vi "Release Session.vi"(0 "Session Handle":T1, 11 "error in (no error)":errorcluster, 13 "force destroy? (F)":bool) -> (15 "error out":errorcluster)   [LabVIEW 2015, in "Circular Buffer.lvclass"]
doc: "Releases an obtained reference to the session"
uses:
  Circular Buffer.lvclass
  Typedefs/Session Handle.ctl
  <userlib>/_Session Fwk/Session - Root.lvclass
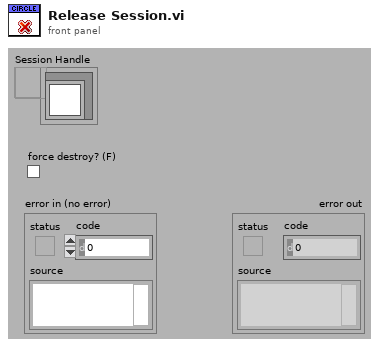
[diagram p1: front panel]
types:
  T1 = typedef "Circular Buffer.lvclass/Session Handle.ctl" = refnum<data-value>
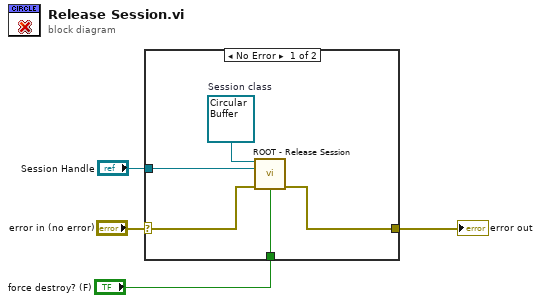
[diagram p0: block diagram]
diagram:
  n1 = case shown="No Error" "error in (no error)" {
    selector: "error in (no error)" -> [w8 w10]
    tunnel: [w7 w10] -> w3
    tunnel: "Session Handle" -> [w9 _]
    tunnel: "force destroy? (F)" -> [w5 _]
    frame No Error {
      w6 = refnum<class "Circular Buffer.lvclass"> refnum  # Session class
      n2 = call <userlib>:"ROOT - Release Session.vi"("OBJ - Session in"=w6, "Session Handle in"=w9, "error in (no error)"=w8, "force destroy? (F)"=w5) -> ("error out"=w7:errorcluster)  [unwired: 9 in, 2 out]
    }
    frame Error {
    }
  }
  "error out" <- w3
